vi "U32toRgba.vi"(11 "U32":u32) -> (3 "Rgba":T1)   [LabVIEW 2020, in "OpenLvVision_Image.lvlib" / "DataAccess.lvlib"]
doc: "Convert an number into an cluster"
uses:
  DataAccess.lvlib
  TypeDef/RgbaU32.ctl
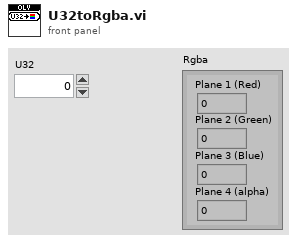
[diagram p1: front panel]
types:
  T1 = typedef "OpenLvVision_Image.lvlib/DataAccess.lvlib/RgbaU32.ctl" = cluster{"Plane 1 (Red)":u8, "Plane 2 (Green)":u8, "Plane 3 (Blue)":u8, "Plane 4 (alpha)":u8}
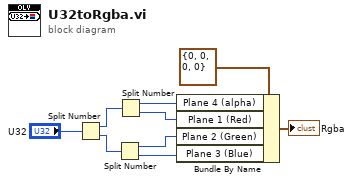
[diagram p0: block diagram]
diagram:
  n1 = Split Number(x="U32") -> (hi(x)=w8:u16, lo(x)=w7:u16)
  n2 = Split Number(x=w7) -> (hi(x)=w2:u8, lo(x)=w4:u8)
  n3 = Split Number(x=w8) -> (hi(x)=w3:u8, lo(x)=w1:u8)
  n4 = Bundle By Name(cluster=T1 {"Plane 1 (Red)"=0, "Plane 2 (Green)"=0, "Plane 3 (Blue)"=0, "Plane 4 (alpha)"=0} ("Color"), "Plane 4 (alpha)"=w3, "Plane 1 (Red)"=w1, "Plane 2 (Green)"=w2, "Plane 3 (Blue)"=w4) -> (→"Rgba":T1)
